vi "configure.vi"(8 "error in (no error)":errorcluster, 9 "write enable":bool=TRUE, 11 "SMSD in":refnum<class "SMSD.lvclass">) -> (0 "error out":errorcluster, 3 "SMSD out":refnum<class "SMSD.lvclass">)   [LabVIEW 2021, in "SMSD.lvclass"]
uses:
  SMSD.lvclass
  SMSD.lvclass/SMSD.ctl
  Data Unit/SMSD Data Unit/ERROR_OR_COMMANT_Type.ctl
  Data Unit/SMSD Data Unit/SMSD Data Unit.lvclass
  Network Protocol/SMSD Master/SMSD Master.lvclass
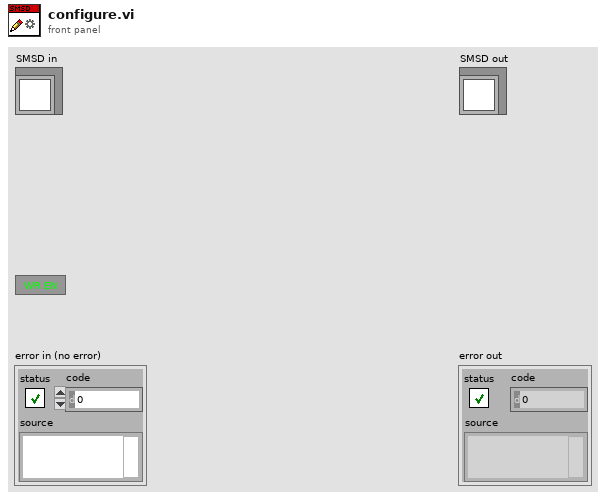
[diagram p1: front panel]
types:
  T1 = enum8{"CMD_PowerSTEP01_END", "CMD_PowerSTEP01_GET_SPEED", "CMD_PowerSTEP01_STATUS_IN_EVENT", "CMD_PowerSTEP01_SET_MODE", "CMD_PowerSTEP01_GET_MODE", "CMD_PowerSTEP01_SET_MIN_SPEED", "CMD_PowerSTEP01_SET_MAX_SPEED", "CMD_PowerSTEP01_SET_ACC", "CMD_PowerSTEP01_SET_DEC", "CMD_PowerSTEP01_SET_FS_SPEED", "CMD_PowerSTEP01_SET_MASK_EVENT", "CMD_PowerSTEP01_GET_ABS_POS", "CMD_PowerSTEP01_GET_EL_POS", "CMD_PowerSTEP01_GET_STATUS_AND_CLR", "CMD_PowerSTEP01_RUN_F", "CMD_PowerSTEP01_RUN_R", "CMD_PowerSTEP01_MOVE_F", "CMD_PowerSTEP01_MOVE_R", "CMD_PowerSTEP01_GO_TO_F", "CMD_PowerSTEP01_GO_TO_R", "CMD_PowerSTEP01_GO_UNTIL_F", "CMD_PowerSTEP01_GO_UNTIL_R", "CMD_PowerSTEP01_SCAN_ZERO_F", "CMD_PowerSTEP01_SCAN_ZERO_R", "CMD_PowerSTEP01_SCAN_LABEL_F", "CMD_PowerSTEP01_SCAN_LABEL_R", "CMD_PowerSTEP01_GO_ZERO", "CMD_PowerSTEP01_GO_LABEL", "CMD_PowerSTEP01_GO_TO", "CMD_PowerSTEP01_RESET_POS", "CMD_PowerSTEP01_RESET_POWERSTEP01", "CMD_PowerSTEP01_SOFT_STOP", "CMD_PowerSTEP01_HARD_STOP", "CMD_PowerSTEP01_SOFT_HI_Z", "CMD_PowerSTEP01_HARD_HI_Z", "CMD_PowerSTEP01_SET_WAIT", "CMD_PowerSTEP01_SET_RELE", "CMD_PowerSTEP01_CLR_RELE", "CMD_PowerSTEP01_GET_RELE", "CMD_PowerSTEP01_WAIT_IN0", "CMD_PowerSTEP01_WAIT_IN1", "CMD_PowerSTEP01_GOTO_PROGRAM", "CMD_PowerSTEP01_GOTO_PROGRAM_IF_IN0", "CMD_PowerSTEP01_GOTO_PROGRAM_IF_IN1", "CMD_PowerSTEP01_LOOP_PROGRAM", "CMD_PowerSTEP01_CALL_PROGRAM", "CMD_PowerSTEP01_RETURN_PROGRAM", "CMD_PowerSTEP01_START_PROGRAM_MEM0", "CMD_PowerSTEP01_START_PROGRAM_MEM1", "CMD_PowerSTEP01_START_PROGRAM_MEM2", "CMD_PowerSTEP01_START_PROGRAM_MEM3", "CMD_PowerSTEP01_STOP_PROGRAM_MEM", "CMD_PowerSTEP01_STEP_CLOCK", "CMD_PowerSTEP01_STOP_USB", "CMD_PowerSTEP01_GET_MIN_SPEED", "CMD_PowerSTEP01_GET_MAX_SPEED", "CMD_PowerSTEP01_GET_STACK", "CMD_PowerSTEP01_GOTO_PROGRAM_IF_ZERO", "CMD_PowerSTEP01_GOTO_PROGRAM_IF_IN_ZERO", "CMD_PowerSTEP01_WAIT_CONTINUE", "CMD_PowerSTEP01_SET_WAIT_2", "CMD_PowerSTEP01_SCAN_MARK2_F", "CMD_PowerSTEP01_SCAN_MARK2_R"}
  T2 = typedef "SMSD Data Unit.lvclass/ERROR_OR_COMMANT_Type.ctl" = enum8{"OK", "OK_ACCESS", "ERROR_ACCESS", "ERROR_ACCESS_TIMEOUT", "ERROR_XOR", "ERROR_NO_COMMAND", "ERROR_LEN", "ERROR_RANGE", "ERROR_WRITE", "ERROR_READ", "ERROR_PROGRAMS", "ERROR_WRITE_SETUP", "NO_NEXT", "END_PROGRAMS", "COMMAND_GET_STATUS_IN_EVENT", "COMMAND_GET_MODE", "COMMAND_GET_ABS_POS", "COMMAND_GET_EL_POS", "COMMAND_GET_SPEED", "COMMAND_GET_MIN_SPEED", "COMMAND_GET_MAX_SPEED", "COMMAND_GET_STACK", "STATUS_RELE_SET", "STATUS_RELE_CLR"}
  T3 = cluster{"min_speed":u32, "max_speed":u32, "acc":u32, "dec":u32}
  T4 = typedef "SMSD Data Unit.lvclass/MOTOR_PARAM.ctl" = cluster{"DRIVER_MODE":T5, "MOTOR_Type_42":T6, "MICROSTEPPING":T7, "WORK_CURRENT":T8, "STOP_CURRENT":T9}
  T5 = typedef "SMSD Data Unit.lvclass/DRIVER_MODE.ctl" = enum16{"VOLTAGE", "CURRENT"}
  T6 = typedef "SMSD Data Unit.lvclass/MOTOR_Type_42.ctl" = enum16{"Unknown", "FL42STH33-1334 1.8 deg", "FL42STH33-1334 0.9 deg", "FL42STH38-1206 0.9 deg", "FL42STH38-1684 1.8 deg", "FL42STH38-1684 0.9 deg", "FL42STH47-1206 1.8 deg", "FL42STH47-1684 1.8 deg", "FL42STH47-1684 0.9 deg", "FL42STH60-1206 1.8 deg", "FL42STH60-1206 0.9 deg", "FL57ST41-1564 1.8 deg", "FL57ST76-1006 1.8 deg", "FL57ST76-1506 1.8 deg", "FL57STH41-1006 1.8 deg", "FL57STH41-1006 0.9 deg", "FL57STH41-2804 1.8 deg", "FL57STH41-2804 0.9 deg", "FL57STH51-1006 1.8 deg", "FL57STH51-2804 1.8 deg", "FL57STH51-2804 0.9 deg", "FL57STH56-1006 1.8 deg", "FL57STH56-2006 1.8 deg", "FL57STH56-2804 1.8 deg", "FL57STH76-1006 1.8 deg", "FL57STH76-2804 1.8 deg", "FL57STH76-2804 0.9 deg", "FL60STH65-2008 1.8 deg parallel", "FL60STH65-2008 1.8 deg serial", "FL60STH86-2008 1.8 deg parallel", "FL60STH86-2008 1.8 deg serial", "FL86STH65-2808 1.8 deg parallel", "FL86STH65-2808 1.8 deg serial", "FL86STH80-4208 1.8 deg parallel", "FL86STH80-4208 1.8 deg serial", "FL86STH118-4208 1.8 deg parallel", "FL86STH118-4208 1.8 deg serial", "FL86STH156-4208 1.8 deg parallel", "FL86STH156-4208 1.8 deg serial", "ДШ3934-0,3А", "ДШ2851-0,7А", "ДШ4248-1,7A", "ДШ5776-3,0А", "ДШ57112-3,0А", "ДШ8665-3,0А", "ДШ8682-4,5А"}
  T7 = typedef "SMSD Data Unit.lvclass/MICROSTEPPING.ctl" = enum16{"1", "1/2", "1/4", "1/8", "1/16", "1/32", "1/64", "1/128"}
  T8 = typedef "SMSD Data Unit.lvclass/WORK_CURRENT.ctl" = enum16{"0.0A", "0.1A", "0.2A", "0.3A", "0.4A", "0.5A", "0.6A", "0.7A", "0.8A", "0.9A", "1.0A", "1.1A", "1.2A", "1.3A", "1.4A", "1.5A", "1.6A", "1.7A", "1.8A", "1.9A", "2.0A", "2.1A", "2.2A", "2.3A", "2.4A", "2.5A", "2.6A", "2.7A", "2.8A", "2.9A", "3.0A", "3.1A", "3.2A", "3.3A", "3.4A", "3.5A", "3.6A", "3.7A", "3.8A", "3.9A", "4.0A", "4.1A", "4.2A", "4.3A", "4.4A", "4.5A", "4.6A", "4.7A", "4.8A", "4.9A", "5.0A", "5.1A", "5.2A", "5.3A", "5.4A", "5.5A", "5.6A", "5.7A", "5.8A", "5.9A", "6.0A", "6.1A", "6.2A", "6.3A", "6.4A", "6.5A", "6.6A", "6.7A", "6.8A", "6.9A", "7.0A", "7.1A", "7.2A", "7.3A", "7.4A", "7.5A", "7.6A", "7.7A", "7.8A", "7.9A", "8.0A", "8.1A", "8.2A"}
  T9 = typedef "SMSD Data Unit.lvclass/STOP_CURRENT.ctl" = enum16{"25%", "50%", "75%", "100%"}
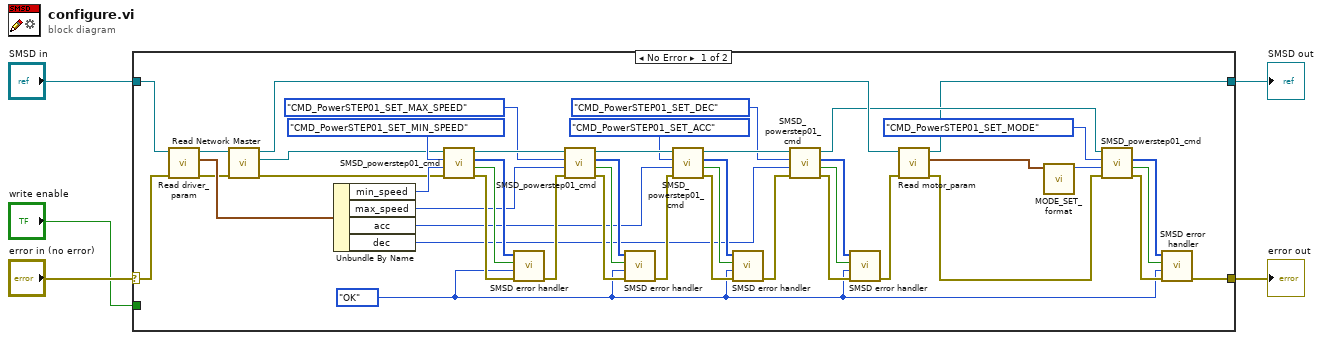
[diagram p0: block diagram]
diagram:
  n1 = case shown="No Error" "error in (no error)" {
    selector: "error in (no error)" -> [w13 w53]
    tunnel: [w18 w53] -> w3
    tunnel: [w6 w52] -> w4
    tunnel: "SMSD in" -> [w14 w52]
    tunnel: "write enable" -> [_ _]
    frame No Error {
      w17 = ERROR_OR_COMMANT_Type."OK" ("coerced x 2")
      n2 = call "Read driver_param.vi"("error in (no error)"=w13, "SMSD in"=w14) -> ("error out"=w12:errorcluster, "Driver_param"=w50:T3, "SMSD out"=w11:refnum<class "SMSD.lvclass">)  [unwired: 7 in]
      n3 = call "Read Network Master.vi"("error in (no error)"=w12, "SMSD in"=w11) -> ("error out"=w9:errorcluster, "TCP Master"=w10:refnum<class "SMSD Master.lvclass">, "SMSD out"=w8:refnum<class "SMSD.lvclass">)  [unwired: 7 in]
      n4 = Unbundle By Name(w50) -> ("min_speed"=w49:u32, "max_speed"=w43:u32, "acc"=w33:u32, "dec"=w25:u32)
      n5 = call "SMSD_powerstep01_cmd.vi"("error in (no error)"=w9, "DATA (0)"=w49, "COMMAND (END)"=T1."CMD_PowerSTEP01_SET_MIN_SPEED", "SMSD in"=w10) -> ("error out"=w47:errorcluster, "PDU valid?"=w46:bool, "data"=w48:u8[], "SMSD out"=w45:refnum<class "SMSD Master.lvclass">)  [unwired: 4 in]
      n6 = call "SMSD error handler.vi"("error in (no error)"=w47, "correct answer (OK)"=w17, "timed out?"=w46, "data"=w48) -> ("error out"=w42:errorcluster)  [unwired: 7 in]
      n7 = call "SMSD_powerstep01_cmd.vi"("error in (no error)"=w42, "DATA (0)"=w43, "COMMAND (END)"=T1."CMD_PowerSTEP01_SET_MAX_SPEED", "SMSD in"=w45) -> ("error out"=w39:errorcluster, "PDU valid?"=w40:bool, "data"=w41:u8[], "SMSD out"=w34:refnum<class "SMSD Master.lvclass">)  [unwired: 4 in]
      n8 = call "SMSD error handler.vi"("error in (no error)"=w39, "correct answer (OK)"=w17, "timed out?"=w40, "data"=w41) -> ("error out"=w35:errorcluster)  [unwired: 7 in]
      n9 = call "SMSD_powerstep01_cmd.vi"("error in (no error)"=w35, "DATA (0)"=w33, "COMMAND (END)"=T1."CMD_PowerSTEP01_SET_ACC", "SMSD in"=w34) -> ("error out"=w38:errorcluster, "PDU valid?"=w37:bool, "data"=w36:u8[], "SMSD out"=w29:refnum<class "SMSD Master.lvclass">)  [unwired: 4 in]
      n10 = call "SMSD error handler.vi"("error in (no error)"=w38, "correct answer (OK)"=w17, "timed out?"=w37, "data"=w36) -> ("error out"=w28:errorcluster)  [unwired: 7 in]
      n11 = call "SMSD_powerstep01_cmd.vi"("error in (no error)"=w28, "DATA (0)"=w25, "COMMAND (END)"=T1."CMD_PowerSTEP01_SET_DEC", "SMSD in"=w29) -> ("error out"=w30:errorcluster, "PDU valid?"=w31:bool, "data"=w32:u8[], "SMSD out"=w7:refnum<class "SMSD Master.lvclass">)  [unwired: 4 in]
      n12 = call "SMSD error handler.vi"("error in (no error)"=w30, "correct answer (OK)"=w17, "timed out?"=w31, "data"=w32) -> ("error out"=w15:errorcluster)  [unwired: 7 in]
      n13 = call "Read motor_param.vi"("error in (no error)"=w15, "SMSD in"=w8) -> ("error out"=w16:errorcluster, "MOTOR_PARAM"=w24:T4, "SMSD out"=w6:refnum<class "SMSD.lvclass">)  [unwired: 7 in]
      n14 = call "MODE_SET_format.vi"("MOTOR_PARAM"=w24) -> ("Data"=w19:u32)  [unwired: 10 in]
      n15 = call "SMSD_powerstep01_cmd.vi"("error in (no error)"=w16, "DATA (0)"=w19, "COMMAND (END)"=T1."CMD_PowerSTEP01_SET_MODE", "SMSD in"=w7) -> ("error out"=w23:errorcluster, "PDU valid?"=w22:bool, "data"=w21:u8[])  [unwired: 4 in, 1 out]
      n16 = call "SMSD error handler.vi"("error in (no error)"=w23, "correct answer (OK)"=w17, "timed out?"=w22, "data"=w21) -> ("error out"=w18:errorcluster)  [unwired: 7 in]
    }
    frame Error {
    }
  }
  "error out" <- w3
  "SMSD out" <- w4
